vi "get channels from scale.vi"(11 "Scale in":T2) -> (3 "Channels":refnum<class "TBM channel.lvclass">[](array[class]))   [LabVIEW 2013, in "Scaling configuration.lvclass"]
uses:
  Scaling configuration.lvclass
  <vilib>/NI/Tag Bus Module Framework/channel/TBM channel.lvclass
  controls/scale data types.ctl
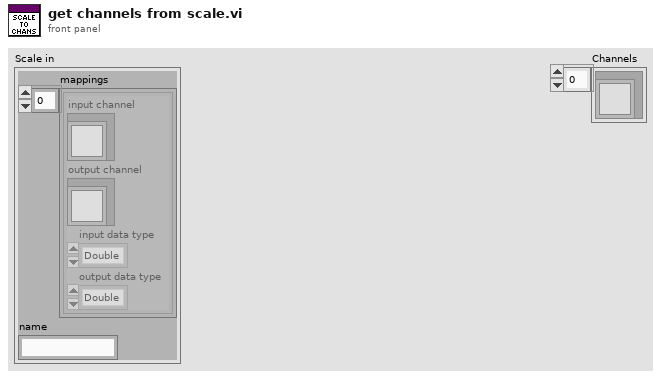
[diagram p1: front panel]
types:
  T1 = typedef "Scaling configuration.lvclass/scale data types.ctl" = enum16{"Double", "Single", "I64", "I32", "I16", "I8", "U64", "U32", "U16", "U8", "Boolean"}
  T2 = cluster{"mappings":cluster{"input channel":refnum<class "TBM channel.lvclass">, "output channel":refnum<class "TBM channel.lvclass">, "input data type":T1, "output data type":T1}[], "name":string}
  T3 = cluster{"input channel":refnum<class "TBM channel.lvclass">, "output channel":refnum<class "TBM channel.lvclass">, "input data type":T1, "output data type":T1}[]
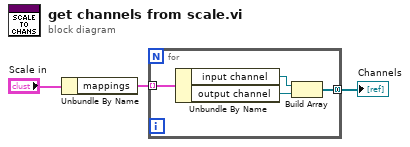
[diagram p0: block diagram]
diagram:
  n1 = Unbundle By Name("Scale in") -> ("mappings"=w3:T3)
  n2 = for {
    tunnel: w3 -> [w7] mode=indexing
    tunnel: [w4] -> w1 mode=concatenating
    n3 = Unbundle By Name(w7) -> ("input channel"=w6:refnum<class "TBM channel.lvclass">, "output channel"=w5:refnum<class "TBM channel.lvclass">)
    n4 = Build Array(w6, w5) -> (w4:refnum<class "TBM channel.lvclass">[])
  }
  "Channels" <- w1
